vi "StripQuality.vi"(3 "Defect Flag array IN":i32[][](array[numeric]), 4 "Strip Length [cm]":dbl=2.386, 6 "Resistance data array":dbl[](array[numeric]), 7 "Capacitance Data Array":dbl[](array[numeric]), 8 "Thresholds:":T1={"Current [nA]"=200.0, "Ccoupl Lo [pF/cm]"=20.0, "Ccoupl Hi [pF/cm]"=33.0, "Rbias Lo [MW]"=1.0, "Rbias Hi [MW]"=2.0}, 9 "Pinhole flag array in":dbl[](array[numeric]), 10 "Channel No. Array":dbl[](array[numeric]), 11 "No of entries":i32) -> (0 "Strip Quality Data":T2 {"pass Rate in %" format="%.2f"}, 1 "Defect code":i32)   [LabVIEW 2013]
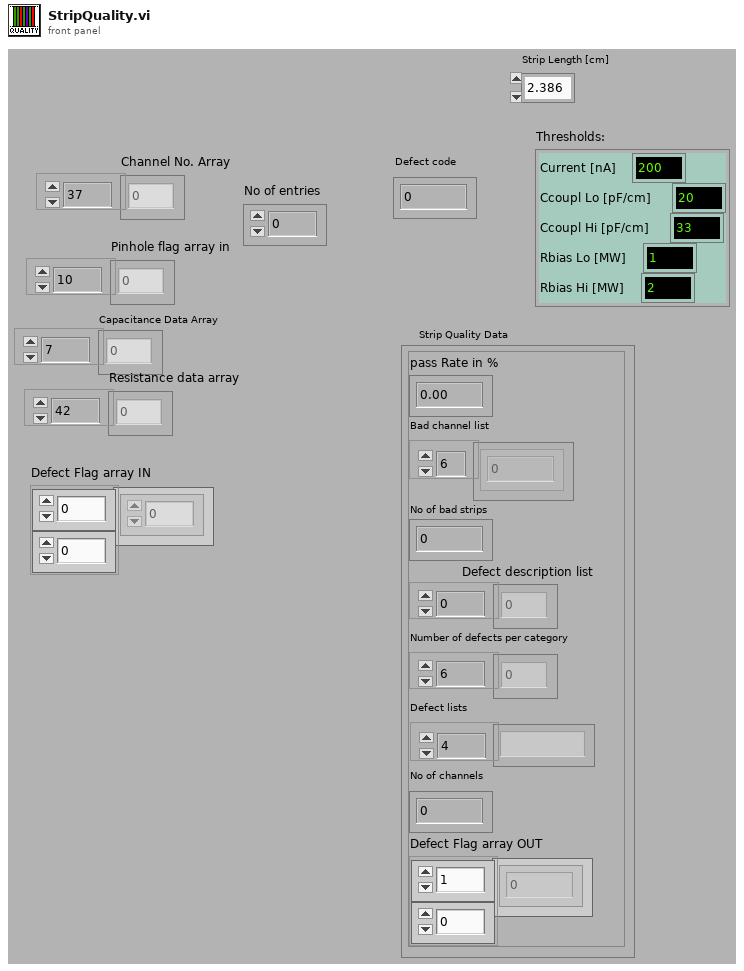
[diagram p1: front panel]
types:
  T1 = cluster{"Current [nA]":dbl, "Ccoupl Lo [pF/cm]":dbl, "Ccoupl Hi [pF/cm]":dbl, "Rbias Lo [MW]":dbl, "Rbias Hi [MW]":dbl}
  T2 = cluster{"pass Rate in %":dbl, "Bad channel list":i32[], "No of bad strips":i32, "Defect description list":i32[], "Number of defects per category":i32[], "Defect lists":string[], "No of channels":i32, "Defect Flag array OUT":i32[][]}
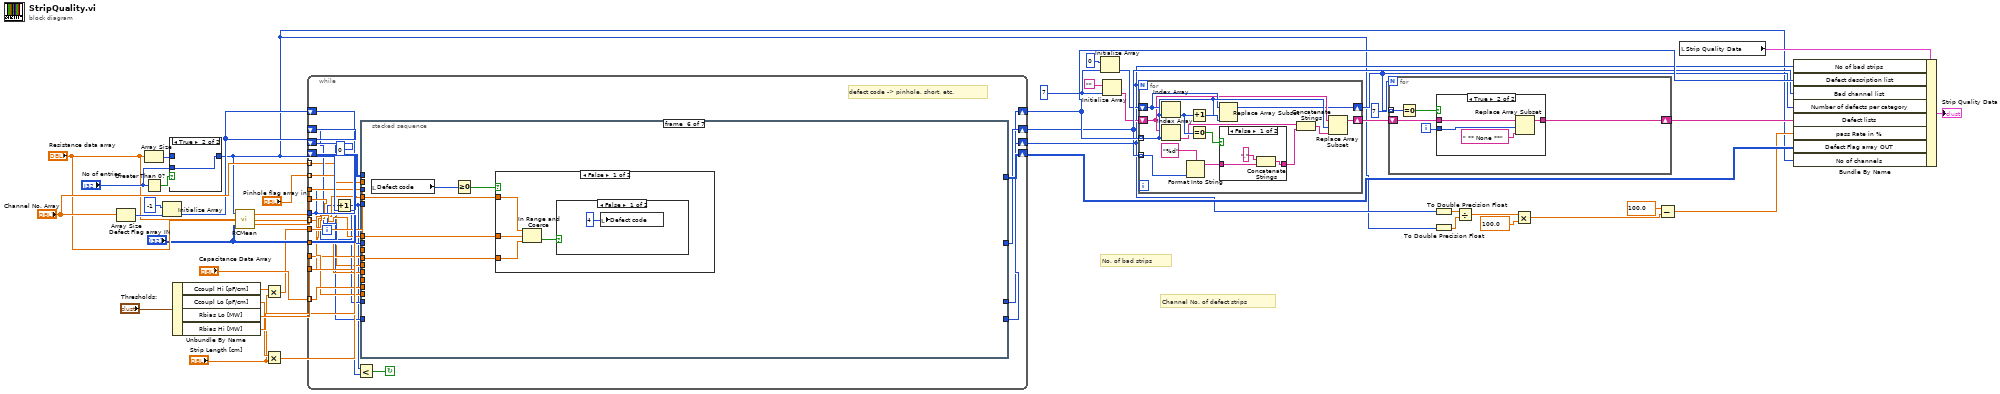
[diagram p0: block diagram]
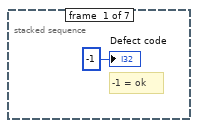
[diagram p2: hidden frame]
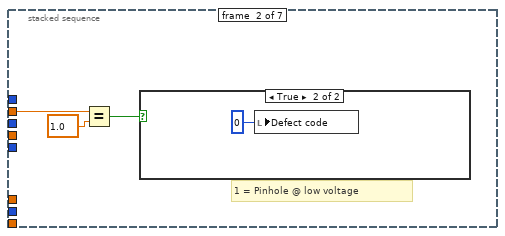
[diagram p3: hidden frame]
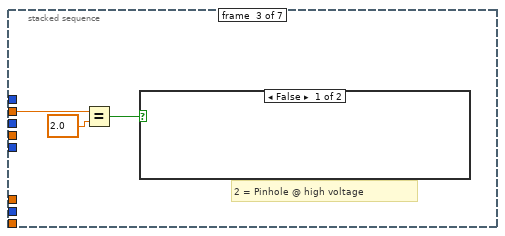
[diagram p5: hidden frame]
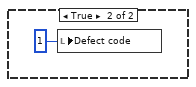
[diagram p6: hidden frame]
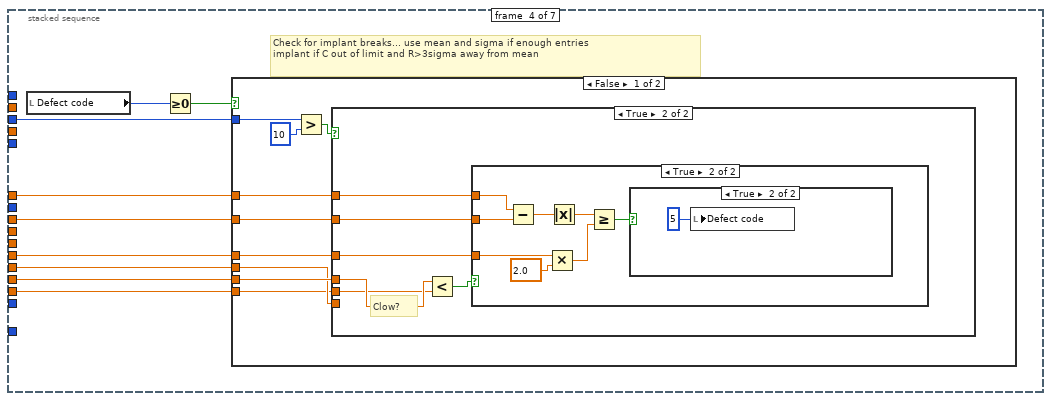
[diagram p7: hidden frame]
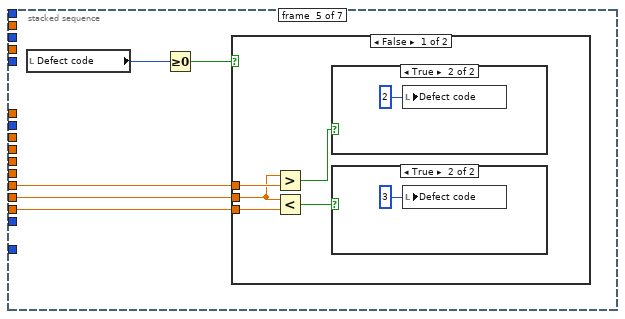
[diagram p12: hidden frame]
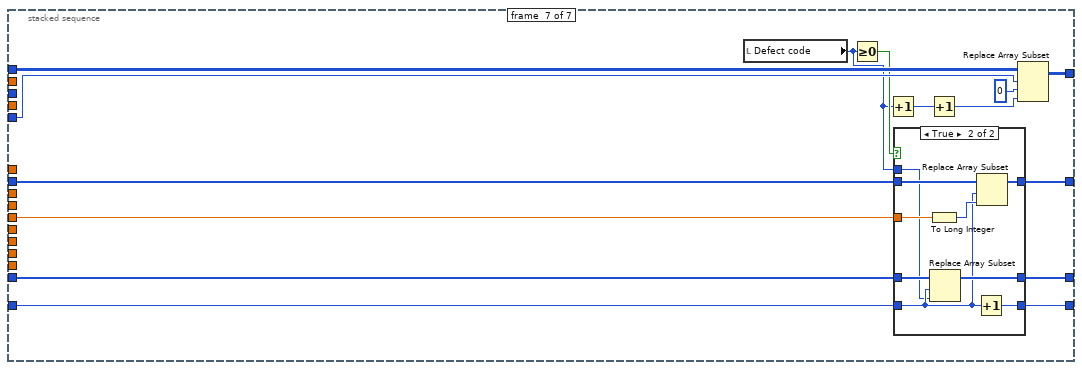
[diagram p18: hidden frame]
diagram:
  w30 = 7 ("Dimension Size")
  # "No. of bad strips"
  # "Channel No. of defect strips"
  n1 = Array Size(array="Channel No. Array") -> (size(s)=w38:i32)
  n2 = Greater Than 0?(x="No of entries") -> (x > 0?=w12:bool)
  n3 = Array Size(array="Resistance data array") -> (size(s)=w9:i32)
  n4 = Initialize Array(-1, w38) -> (w36:i32[])
  n5 = case shown="True" w12 {
    tunnel: "No of entries" -> [_ w47]
    tunnel: [w46 w47] -> w8
    tunnel: w9 -> [w46 _]
    frame False {
    }
    frame True {
    }
  }
  n6 = Unbundle By Name("Thresholds:") -> ("Ccoupl Hi [pF/cm]"=w6:dbl, "Ccoupl Lo [pF/cm]"=w5:dbl, "Rbias Lo [MW]"=w41:dbl, "Rbias Hi [MW]"=w40:dbl)
  n7 = call "RCMean.vi"("Defect Flag array IN"="Defect Flag array IN", "data array in"="Resistance data array", "No of strips"=w8) -> ("standard deviation"=w42:dbl, "mean"=w43:dbl)
  n8 = Multiply(x=w6, y="Strip Length [cm]") -> (x*y=w4:dbl)
  n9 = Multiply(x=w5, y="Strip Length [cm]") -> (x*y=w3:dbl)
  n10 = while {
    shift-left: 0 -> [w53]
    shift-right: [w52] -> w20
    shift-left: w36 -> [w56]
    shift-right: [w51] -> w32
    shift-left: w36 -> [w57]
    shift-right: [w54] -> w31
    shift-left: "Defect Flag array IN" -> [w59]
    shift-right: [w58] -> w21
    tunnel: w40 -> [w60]
    tunnel: w41 -> [w61]
    tunnel: w42 -> [w62]
    tunnel: w43 -> [w63]
    tunnel: "Resistance data array" -> [w64] mode=indexing
    tunnel: w3 -> [w65]
    tunnel: w4 -> [w66]
    tunnel: "Capacitance Data Array" -> [w67] mode=indexing
    tunnel: "Channel No. Array" -> [w55] mode=indexing
    tunnel: "Pinhole flag array in" -> [w68] mode=indexing
    tunnel: w8 -> [w50]
    i -> [w49]
    stop <- w69 continue-if-true
    # "defect code -> pinhole, short, etc."
    n11 = Increment(x=w49) -> (x+1=w48:i32)
    n12 = Less?(x=w48, y=w50) -> (x < y?=w69:bool)
    n13 = stacked-sequence {
      tunnel: w68 -> [_ w73 w77 _ _ _ _]
      tunnel: w50 -> [_ _ _ w85 _ _ _]
      tunnel: w67 -> [_ _ _ w84 w114 _ _]
      tunnel: w66 -> [_ _ _ w83 w113 _ _]
      tunnel: w65 -> [_ _ _ w82 w112 _ _]
      tunnel: w64 -> [_ _ _ w81 _ w126 _]
      tunnel: w63 -> [_ _ _ w80 _ _ _]
      tunnel: w62 -> [_ _ _ w79 _ _ _]
      tunnel: w61 -> [_ _ _ _ _ w125 _]
      tunnel: w60 -> [_ _ _ _ _ w124 _]
      tunnel: w59 -> [_ _ _ _ _ _ w148]
      tunnel: w48 -> [_ _ _ _ _ _ w147]
      tunnel: [_ _ _ _ _ _ w145] -> w58
      tunnel: w57 -> [_ _ _ _ _ _ w144]
      tunnel: w56 -> [_ _ _ _ _ _ w140]
      tunnel: w55 -> [_ _ _ _ _ _ w143]
      tunnel: [_ _ _ _ _ _ w142] -> w54
      tunnel: w53 -> [_ _ _ _ _ _ w139]
      tunnel: [_ _ _ _ _ _ w138] -> w52
      tunnel: [_ _ _ _ _ _ w137] -> w51
      frame #0 {
        # "-1 = ok"
        "Defect code" <- -1 ("Defect code")
      }
      frame #1 {
        # "1 = Pinhole @ low voltage"
        n14 = Equal?(x=w73, y=1.0) -> (x = y?=w71:bool)
        n15 = case shown="True" w71 {
          frame False {
          }
          frame True {
            n16 = local write "Defect code"(0 ("Defect code")) -> ()
          }
        }
      }
      frame #2 {
        # "2 = Pinhole @ high voltage"
        n17 = Equal?(x=w77, y=2.0) -> (x = y?=w75:bool)
        n18 = case shown="False" w75 {
          frame False {
          }
          frame True {
            n19 = local write "Defect code"(1 ("Defect code")) -> ()
          }
        }
      }
      frame #3 {
        # "Check for implant breaks... use mean and sigma if enough entries\nimplant if C out of limit and R>3sigma away from mean"
        n20 = local read "Defect code"() -> (w87:i32)
        n21 = Greater Or Equal To 0?(x=w87) -> (x >= 0?=w86:bool)
        n22 = case shown="False" w86 {
          tunnel: w85 -> [w96 _]
          tunnel: w84 -> [w93 _]
          tunnel: w83 -> [w92 _]
          tunnel: w82 -> [w91 _]
          tunnel: w81 -> [w90 _]
          tunnel: w80 -> [w89 _]
          tunnel: w79 -> [w88 _]
          frame False {
            n23 = Greater?(x=w96, y=10) -> (0:w94:bool)
            n24 = case shown="True" w94 {
              tunnel: w93 -> [_ w102]
              tunnel: w92 -> [_ _]
              tunnel: w91 -> [_ w101]
              tunnel: w90 -> [_ w99]
              tunnel: w89 -> [_ w98]
              tunnel: w88 -> [_ w97]
              frame False {
              }
              frame True {
                # "Clow?"
                n25 = Less?(x=w102, y=w101) -> (x < y?=w100:bool)
                n26 = case shown="True" w100 {
                  tunnel: w99 -> [_ w110]
                  tunnel: w98 -> [_ w109]
                  tunnel: w97 -> [_ w107]
                  frame False {
                  }
                  frame True {
                    n27 = Subtract(x=w110, y=w109) -> (x-y=w108:dbl)
                    n28 = Multiply(x=w107, y=2.0) -> (x*y=w104:dbl)
                    n29 = Absolute Value(x=w108) -> (abs(x)=w105:dbl)
                    n30 = Greater Or Equal?(x=w105, y=w104) -> (x >= y?=w103:bool)
                    n31 = case shown="True" w103 {
                      frame False {
                      }
                      frame True {
                        n32 = local write "Defect code"(5 ("Defect code")) -> ()
                      }
                    }
                  }
                }
              }
            }
          }
          frame True {
          }
        }
      }
      frame #4 {
        n33 = local read "Defect code"() -> (w116:i32)
        n34 = Greater Or Equal To 0?(x=w116) -> (x >= 0?=w115:bool)
        n35 = case shown="False" w115 {
          tunnel: w114 -> [w119 _]
          tunnel: w113 -> [w121 _]
          tunnel: w112 -> [w118 _]
          frame False {
            n36 = Greater?(x=w119, y=w121) -> (0:w120:bool)
            n37 = Less?(x=w119, y=w118) -> (x < y?=w117:bool)
            n38 = case shown="True" w120 {
              frame False {
              }
              frame True {
                n39 = local write "Defect code"(2 ("Defect code")) -> ()
              }
            }
            n40 = case shown="True" w117 {
              frame False {
              }
              frame True {
                n41 = local write "Defect code"(3 ("Defect code")) -> ()
              }
            }
          }
          frame True {
          }
        }
      }
      frame #5 {
        n42 = local read "Defect code"() -> (w128:i32)
        n43 = Greater Or Equal To 0?(x=w128) -> (x >= 0?=w127:bool)
        n44 = case shown="False" w127 {
          tunnel: w126 -> [w132 _]
          tunnel: w125 -> [w131 _]
          tunnel: w124 -> [w130 _]
          frame False {
            n45 = In Range and Coerce(upper limit=w130, x=w132, lower limit=w131) -> (In Range?=w129:bool)  [unwired: 1 out]
            n46 = case shown="False" w129 {
              frame False {
                n47 = local write "Defect code"(4 ("Defect code")) -> ()
              }
              frame True {
              }
            }
          }
          frame True {
          }
        }
      }
      frame #6 {
        n48 = local read "Defect code"() -> (w134:i32)
        n49 = Greater Or Equal To 0?(x=w134) -> (x >= 0?=w141:bool)
        n50 = Increment(x=w134) -> (x+1=w135:i32)
        n51 = case shown="True" w141 {
          tunnel: w144 -> [w151 w160]
          tunnel: w143 -> [_ w158]
          tunnel: [w151 w157] -> w142
          tunnel: w140 -> [w150 w156]
          tunnel: w139 -> [w149 w153]
          tunnel: [w149 w155] -> w138
          tunnel: [w150 w154] -> w137
          tunnel: w134 -> [_ w152]
          frame False {
          }
          frame True {
            n52 = To Long Integer(number=w158) -> (32bit integer=w159:i32)
            n53 = Replace Array Subset(array=w156, new element=w152, index=w153) -> (w154:i32[])
            n54 = Increment(x=w153) -> (x+1=w155:i32)
            n55 = Replace Array Subset(array=w160, new element=w159, index=w153) -> (w157:i32[])
          }
        }
        n56 = Increment(x=w135) -> (x+1=w136:i32)
        n57 = Replace Array Subset(array=w148, new element=w136, index (row)=w147, index (col)=0 ("Index")) -> (w145:i32[][])
      }
    }
  }
  n58 = Initialize Array(0, w30) -> (w28:i32[])
  n59 = Initialize Array("", w30) -> (w27:string[])
  n60 = for {
    N: w20 -> [_]
    tunnel: w32 -> [w165] mode=indexing
    tunnel: w31 -> [w170] mode=indexing
    shift-right: [w162] -> w25
    shift-left: w28 -> [w164]
    shift-right: [w161] -> w24
    shift-left: w27 -> [w163]
    n61 = Index Array(array=w164, index=w165) -> (element=w173:i32)
    n62 = Index Array(array=w163, index=w165) -> (element=w168:string)
    n63 = Format Into String(format string="%d" ("Format String"), w170) -> (resulting string=w169:string)  [unwired: 2 in, 1 out]
    n64 = Increment(x=w173) -> (x+1=w174:i32)
    n65 = Equal To 0?(x=w173) -> (x = 0?=w172:bool)
    n66 = Replace Array Subset(array=w164, new element=w174, index=w165) -> (w162:i32[])
    n67 = case shown="False" w172 {
      tunnel: w169 -> [w175 w178]
      tunnel: [w177 w178] -> w167
      frame False {
        n68 = Concatenate Strings(",", w175) -> (w177:string)
      }
      frame True {
      }
    }
    n69 = Concatenate Strings(w168, w167) -> (w166:string)
    n70 = Replace Array Subset(array=w163, new element=w166, index=w165) -> (w161:string[])
  }
  n71 = for {
    N: 7 -> [_]
    tunnel: w25 -> [w183] mode=indexing
    shift-right: [w179] -> w23
    shift-left: w24 -> [w181]
    i -> [w180]
    n72 = Equal To 0?(x=w183) -> (x = 0?=w182:bool)
    n73 = case shown="True" w182 {
      tunnel: w181 -> [w184 w188]
      tunnel: w180 -> [_ w186]
      tunnel: [w184 w185] -> w179
      frame False {
      }
      frame True {
        n74 = Replace Array Subset(array=w188, new element=" ** None **" ("Element Data"), index=w186) -> (w185:string[])
      }
    }
  }
  n75 = To Double Precision Float(number=w20) -> (double precision float=w19:dbl)
  n76 = To Double Precision Float(number=w8) -> (double precision float=w18:dbl)
  n77 = Divide(x=w19, y=w18) -> (x/y=w17:dbl)
  n78 = Multiply(x=w17, y=100.0) -> (x*y=w14:dbl)
  n79 = Subtract(x=100.0, y=w14) -> (x-y=w13:dbl)
  n80 = local read "Strip Quality Data"() -> (w34:T2)
  n81 = Bundle By Name(cluster=w34, "No of bad strips"=w20, "Defect description list"=w32, "Bad channel list"=w31, "Number of defects per category"=w25, "Defect lists"=w23, "pass Rate in %"=w13, "Defect Flag array OUT"=w21, "No of channels"=w8) -> (→"Strip Quality Data":T2)
